vi "Window-ROI scrolling window.vi"() -> ()   [LabVIEW 2020]
uses:
  Typedefs/Get-Set-Clear Control.ctl
  Global variables/gl_Functional Imaging-Global variables.vi
  Global Variables/General Globals.vi
panel:
  in  "Scrollbar":i32(c297)
  out "Selected ROI":i32 caption="Selected:" format="ROI %.0f"
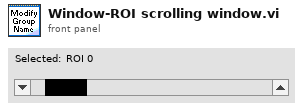
[diagram p1: front panel]
types:
  T1 = typedef "Get-Set-Clear Control.ctl" = enum16{"Get", "Set", "Clear"}
  T2 = typedef "Functional Imging UI Refs.ctl" = cluster{"Menu ref":refnum<k9>, "Image control":refnum<vi>, "VI ref":refnum<vi>, "XGrapher":refnum<vi>, "Smoothing":refnum<vi>, "POI Averaging":refnum<vi>, "Normalize":refnum<vi>, "POI data points in each trial":refnum<vi>, "Channel":refnum<vi>, "Experiment data folder path":refnum<vi>, "[ROI vis]":refnum<vi>, "[Groups] visbl":T3, "Group Name":refnum<vi>, "POI index":refnum<vi>, "Trial No.":refnum<vi>, "Intensity Zoom":refnum<vi>, "Trial Cursor Enabled":refnum<vi>, "Number of Trials (ind 1)":refnum<vi>, "Number of Trials (ind 2)":refnum<vi>, "MiniScans Available":refnum<vi>, "POI Available":refnum<vi>, "Defer graph updates":refnum<vi>, "Waveform selector":refnum<vi>, "#of selected POI":refnum<vi>, "#of selected MiniScans":refnum<vi>, "#of selected groups":refnum<vi>, "Max Z-Projection":refnum<vi>, "Z-Plane Selector":refnum<vi>, "Index of miniscan point to visualise":refnum<vi>, "ROI vis. mode":refnum<vi>, "Total # of points":refnum<vi>, "Index of group clicked on":refnum<vi>, "Pane 1":refnum<vi>, "Pane 2":refnum<vi>, "Pane 3":refnum<vi>, "Pane 4":refnum<vi>, "Pane 5":refnum<vi>, "Pane 6":refnum<vi>, "Deselect all ROI":refnum<vi>, "Deselect all groups":refnum<vi>}
  T3 = typedef "Groups array referecne.ctl" = refnum<vi>
  T4 = typedef "ROI selector array-ROI vis.ctl" = T5[]
  T5 = typedef "Interface-ROI selection cluster.ctl" = cluster{"ROI number":i32, "ROI ID":T6, "Visibility":bool}
  T6 = typedef "ROI ID Enum.ctl" = enum16{"Point", "MiniScan", "Comp. MiniScan", "Rectangle", "Comp. volume", "Arb. plane point", "None"}
  T7 = typedef "ROI group info cluster.ctl" = cluster{"Group name":string, "# ROI in group":i32, "ROI numbers in group":i32[], "Group region specifier cluster":T8}
  T8 = typedef "ROI Descriptor" = cluster{"Global Rectangle":i32[], "Contours":cluster{"ID":enum32{"External", "Internal"}, "Type":u32, "Coordinates":i32[]}[]}
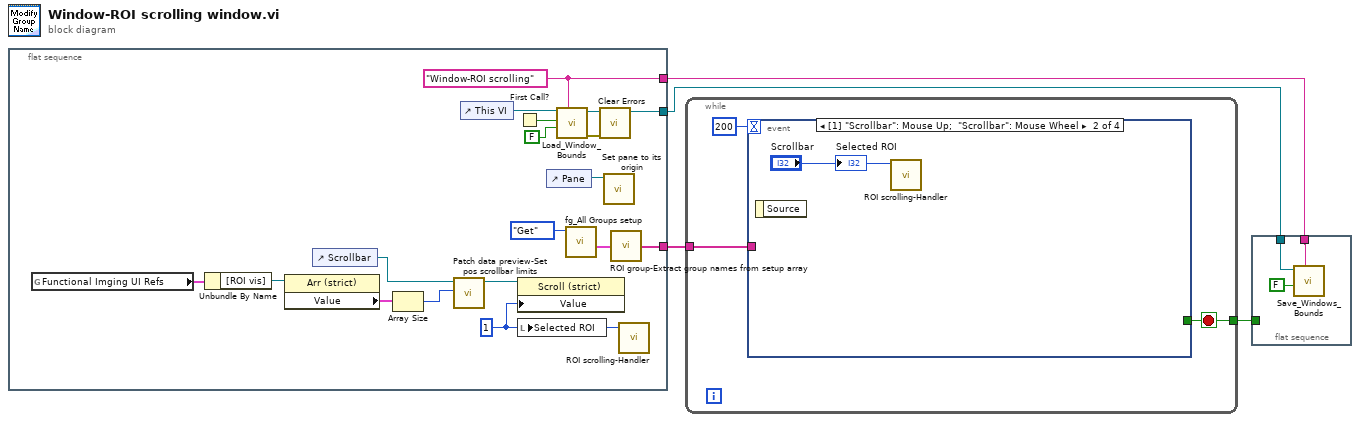
[diagram p0: block diagram]
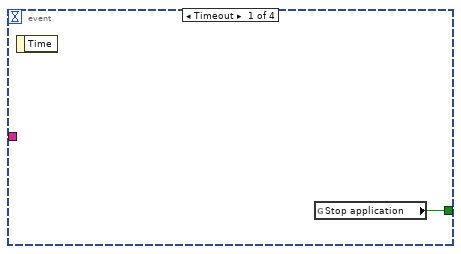
[diagram p2: hidden frame]
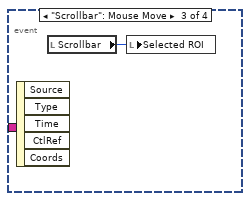
[diagram p3: hidden frame]
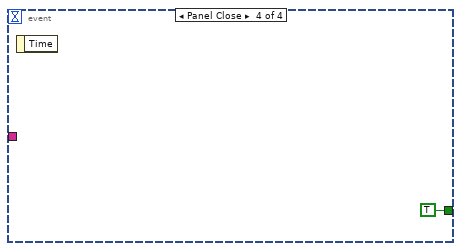
[diagram p4: hidden frame]
diagram:
  n1 = flat-sequence {
    tunnel: [w17] -> w4
    tunnel: [w16] -> w3
    tunnel: [w12] -> w2
    frame #0 {
      w5 = 1 ("Slider")
      w17 = "Window-ROI scrolling" ("Window Name (i.e. Key)")
      n2 = global read "gl_Functional Imaging-Global variables.vi" "Functional Imging UI Refs"() -> (w9:T2)
      n3 = Unbundle By Name(w9) -> ("[ROI vis]"=w10:refnum<vi>)
      n4 = property class="Arr (strict)"(reference=w10) -> ("Value"=w11:T4)  [unwired: 1 in, 2 out]
      n5 = control-ref of="Scrollbar"() -> (w8:refnum<vi>)
      n6 = Array Size(array=w11) -> (size(s)=w7:i32)
      n7 = call "Patch data preview-Set pos scrollbar limits.vi"("Last cycle's number"=w7, "Scrollbar"=w8) -> ("Scrollbar"=w6:refnum<vi>)  [unwired: 8 in, 1 out]
      n8 = control-ref of="This VI"() -> (w15:refnum<vi>)
      n9 = First Call?() -> (First Call?: T/F=w19:bool)
      n10 = property class="Scroll (strict)"(reference=w6, "Value"=w5) -> ()  [unwired: 1 in, 2 out]
      n11 = local write "Selected ROI"(w5) -> ()
      n12 = control-ref of="Pane"() -> (w21:refnum<vi>)
      n13 = call "Load_Window_Bounds.vi"("Window Name (i.e. Key)"=w17, "Disable"=FALSE, "First Call"=w19, "Window VI's Ref"=w15) -> ("error out"=w18:errorcluster, "reference out"=w16:refnum<vi>)  [unwired: 4 in, 2 out]
      n14 = call "fg_All Groups setup.vi"("Function"=Get-Set-Clear_Control."Get") -> ("Groups setup out"=w14:T7[])  [unwired: 9 in, 1 out]
      n15 = call <vilib>:"Clear Errors.vi"("error in (no error)"=w18) -> ()  [unwired: 5 in, 2 out]
      n16 = call <userlib>:"Set pane to its origin.vi"("Pane Reference"=w21) -> ()  [unwired: 9 in, 2 out]
      n17 = call "ROI group-Extract group names from setup array.vi"("Groups setup"=w14) -> ("Group Names Array"=w12:string[])
      n18 = call "ROI scrolling-Handler.vi"("ROI number"=w5) -> ()  [unwired: 11 in]
    }
  }
  n19 = while {
    tunnel: [w24] -> w1
    tunnel: w2 -> [w22]
    stop <- w24 stop-if-true
    n20 = event shown="[1] \"Scrollbar\": Mouse Up;  \"Scrollbar\": Mouse Wheel" {
      selector: _ -> [_ _ _ _]
      dyn-events: _ -> [_ _ _ _]
      timeout: 200 -> [_ _ _ _]
      tunnel: [w25 _ _ TRUE] -> w24
      tunnel: w22 -> [_ _ _ _]
      event Timeout {
        n21 = event-data() -> ()  [unwired: 1 in, 1 out]
        n22 = global read "General Globals.vi" "Stop application"() -> (w25:bool)
      }
      event "Scrollbar": Mouse Up; "Scrollbar": Mouse Wheel {
        n23 = event-data() -> ()  [unwired: 1 in, 1 out]
        n24 = call "ROI scrolling-Handler.vi"("ROI number"="Scrollbar") -> ()  [unwired: 11 in]
        "Selected ROI" <- "Scrollbar"
      }
      event "Scrollbar": Mouse Move {
        n25 = event-data() -> ()  [unwired: 1 in, 5 out]
        n26 = local read "Scrollbar"() -> (w27:i32)
        n27 = local write "Selected ROI"(w27) -> ()
      }
      event Panel Close {
        n28 = event-data() -> ()  [unwired: 1 in, 1 out]
      }
    }
  }
  n29 = flat-sequence {
    tunnel: w4 -> [w30]
    tunnel: w3 -> [w31]
    tunnel: w1 -> [_]
    frame #0 {
      n30 = call "Save_Windows_Bounds.vi"("Window Name (i.e. Key)"=w30, "Front Panel Window:Open"=FALSE, "Window VI's Ref"=w31) -> ()  [unwired: 8 in, 1 out]
    }
  }
